vi "test.ingest_csv 2.vi"   [LabVIEW 2020]
uses:
  Nominal Client/Nominal Client.lvclass
  timestampMetadata/timestampMetadata.lvclass
  f68fde30-30e4-4b08-97bf-6f7da0132bc9.vi
  datasources/source/source.lvclass
  datasources/source/create_s3.vi
  datasources/target/target.lvclass
  datasources/target/create_new.vi
  nominal types/channelConfig/channelConfig.lvclass
  datasources/dataset/dataset.lvclass
  d999190f-fee9-49b3-afb9-f232f2b660b8.vi
  Nominal Client/ingest_csv.vi
  nominal types/properties/properties.lvclass
  ts.iso8601/build.iso8601.vi
  ts.iso8601/ts.iso8601.lvclass
  datasources/s3/s3.lvclass
  C:/code/labview-client/lv_src/Nominal Client/datasources/source/source.lvclass
  C:/code/labview-client/lv_src/Nominal Client/datasources/payload/payload.lvclass
  C:/code/labview-client/lv_src/Nominal Client/datasources/s3/s3.lvclass
types:
  T1 = cluster{"dataset":refnum<class "dataset.lvclass">, "channelConfig":refnum<class "channelConfig.lvclass">}
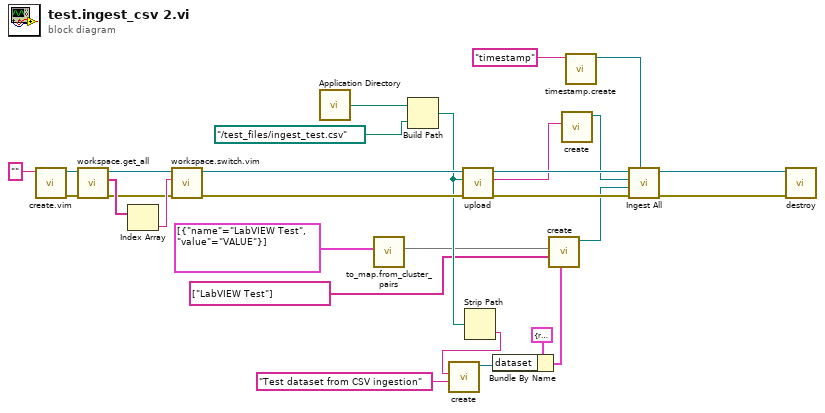
[diagram p0: block diagram]
diagram:
  n1 = call "create.vim"("API Token (string or path)"="") -> ("error out"=w14:errorcluster, "Nominal Client"=w18:refnum<class "Nominal Client.lvclass">)  [unwired: 9 in]
  n2 = call "workspace.get_all.vi"("error in"=w14, "Nominal Client in"=w18) -> ("error out"=w13:errorcluster, "Workspace RIDs"=w16:string[], "Nominal Client out"=w17:refnum<class "Nominal Client.lvclass">)  [unwired: 5 in, 2 out]
  n3 = Index Array(array=w16) -> (element=w15:string)  [unwired: 1 in]
  n4 = call "workspace.switch.vim"("error in"=w13, "Workspace RID (string or path)"=w15, "Nominal Client in"=w17) -> ("error out"=w12:errorcluster, "Nominal Client out"=w11:refnum<class "Nominal Client.lvclass">)  [unwired: 7 in]
  n5 = call <vilib>:"Application Directory.vi"() -> ("Application Directory"=w21:path)
  n6 = call "to_map.from_cluster_pairs.vi"("properties (cluster pairs)"=cluster{"name":string, "value":string}[] [{"name"="LabVIEW Test", "value"="VALUE"}] ("properties")) -> ("properties (map)"=w1:map{string, string})  [unwired: 10 in]
  n7 = Build Path(base path=w21, name or relative path=path "../test_files/ingest_test.csv") -> (appended path=w6:path)
  n8 = call "upload.vi"("error in"=w12, "File"=w6, "Nominal Client in"=w11) -> ("error out"=w26:errorcluster, "Path to S3 File"=w25:string, "Nominal Client out"=w27:refnum<class "Nominal Client.lvclass">)  [unwired: 6 in]
  n9 = Strip Path(path=w6) -> (name=w5:string)  [unwired: 1 out]
  n10 = call "create.vi"("Description"="Test dataset from CSV ingestion", "Name"=w5) -> ("dataset"=w8:refnum<class "dataset.lvclass">)  [unwired: 9 in]
  n11 = Bundle By Name(cluster=T1 {"dataset"=refnum, "channelConfig"=refnum} ("Optional"), "dataset"=w8) -> (w9:T1)
  n12 = call-poly "create.vi"("Optional"=w9, "Labels"=string[] ["LabVIEW Test"] ("labels"), "Properties"=w1) -> ("New Target"=w23:refnum<class "target.lvclass">)  [unwired: 8 in]
  n13 = call-poly "create.vi"("Path"=w25) -> ("source"=w24:refnum<class "s3.lvclass">)  [unwired: 10 in]
  n14 = call-poly "timestamp.create.vi"("seriesName"="timestamp") -> ("Timestamp Metadata"=w4:refnum<class "timestampMetadata.lvclass">)  [unwired: 10 in]
  n15 = call-poly "Ingest All.vi"("timestampMetadata"=w4, "error in"=w26, "Target"=w23, "Source"=w24, "Nominal Client in"=w27) -> ("error out"=w28:errorcluster, "Nominal Client out"=w29:refnum<class "Nominal Client.lvclass">)  [unwired: 3 in, 2 out]
  n16 = call "destroy.vi"("error in"=w28, "Nominal Client"=w29) -> ()  [unwired: 9 in, 1 out]
